vi "set_dataConverter.vi"(0 "HGV_PVBase":refnum<class "HGF_PVBase.lvclass">, 2 "HGF_PVDataConverter":refnum<class "HGF_PVDataConverter.lvclass">, 5 "error in (no error)":errorcluster) -> (14 "dup HGV_PVBase":refnum<class "HGF_PVBase.lvclass">, 19 "error out":errorcluster)   [LabVIEW 2014, in "HGF_BaseClasses.lvlib" / "HGF_PVBase.lvclass"]
doc: "Set DataConverter object."
uses:
  HGF_PVBase.lvclass
  HGF_PVDataConverter/HGF_PVDataConverter.lvclass
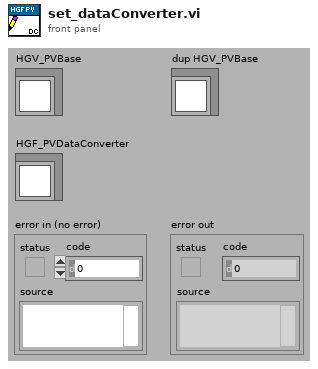
[diagram p1: front panel]
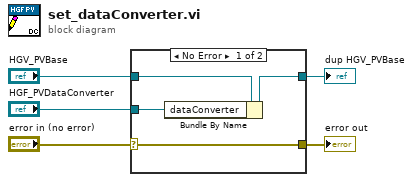
[diagram p0: block diagram]
diagram:
  n1 = case shown="No Error" "error in (no error)" {
    selector: "error in (no error)" -> [w9 w10]
    tunnel: [w9 w10] -> w4
    tunnel: [w7 w11] -> w2
    tunnel: "HGV_PVBase" -> [w8 w11]
    tunnel: "HGF_PVDataConverter" -> [w6 _]
    frame No Error {
      n2 = Bundle By Name(cluster=w8, "dataConverter"=w6) -> (w7:refnum<class "HGF_PVBase.lvclass">)
    }
    frame Error {
    }
  }
  "error out" <- w4
  "dup HGV_PVBase" <- w2
